vi "FitVItoLargestDecBounds.vi"(8 "error in (no error)":errorcluster, 11 "VI Ref (calling VI)":refnum<vi>) -> (0 "error out":errorcluster, 2 "content size":T1, 3 "dup VI Ref":refnum<vi>)   [LabVIEW 2021, in "TipStripOOPanelExample.lvlib" / "TipPanelExample.lvclass"]
uses:
  TipPanelExample.lvclass
  <vilib>/Utility/miscctls.llb/LVBoundsTypeDef.ctl
  TipPanelExample.lvclass/TipPanelExample.ctl
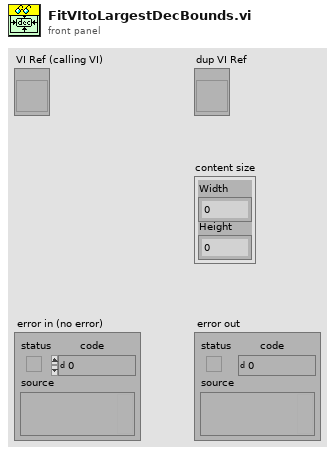
[diagram p1: front panel]
types:
  T1 = typedef "LVBoundsTypeDef.ctl" = cluster{"Width":u32, "Height":u32}
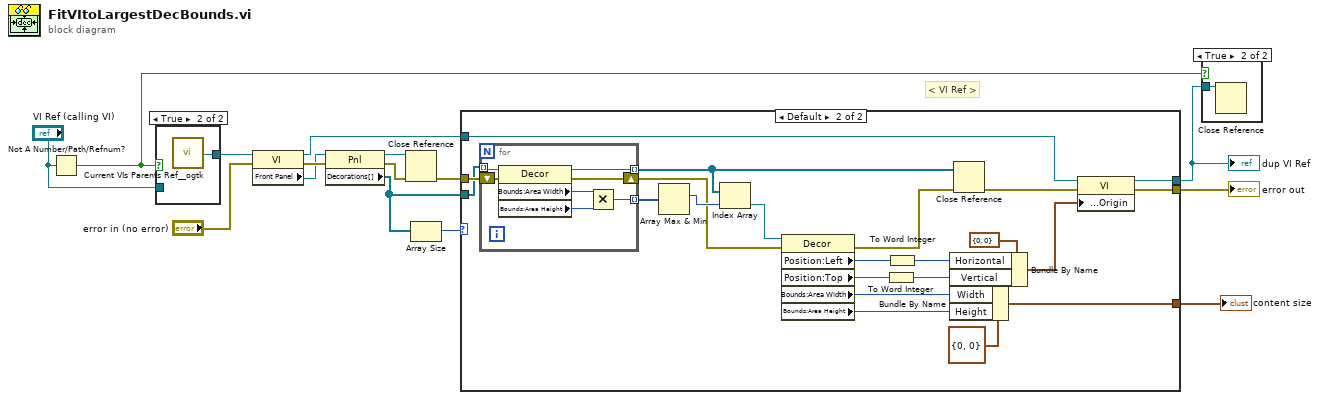
[diagram p0: block diagram]
diagram:
  # "< VI Ref >"
  n1 = Not A Number/Path/Refnum?(number/path/refnum="VI Ref (calling VI)") -> (NaN/Path/Refnum?=w3:bool)
  n2 = case shown="True" w3 {
    tunnel: [w16 w17] -> w4
    tunnel: "VI Ref (calling VI)" -> [w16 _]
    frame False {
    }
    frame True {
      n3 = call <userlib>:"Current VIs Parents Ref__ogtk.vi"() -> ("Calling VI's Reference"=w17:refnum<vi>)  [unwired: 2 in]
    }
  }
  n4 = property on="Property Node" class="VI"(reference=w4, error in="error in (no error)") -> (reference out=w15:refnum<vi>, error out=w13:errorcluster, "Front Panel"=w10:refnum<vi>)
  n5 = property on="Property Node" class="Pnl"(reference=w10, error in=w13) -> (reference out=w14:refnum<vi>, error out=w12:errorcluster, "Decorations[]"=w7:refnum<vi>[])
  n6 = Close Reference(reference=w14, error in (no error)=w12) -> (error out=w9:errorcluster)
  n7 = Array Size(array=w7) -> (size(s)=w6:i32)
  n8 = case shown="Default" w6 {
    tunnel: w15 -> [w19 w41]
    tunnel: w9 -> [w18 w36]
    tunnel: [w18 w24] -> w8
    tunnel: [w19 w25] -> w2
    tunnel: w7 -> [_ w28]
    tunnel: [_ w20] -> w1
    frame 0 {
    }
    frame Default {
      n9 = for {
        tunnel: w28 -> [w48] mode=indexing
        tunnel: [w45] -> w35 mode=indexing
        shift-right: [w43] -> w31
        shift-left: w36 -> [w44]
        tunnel: [w42] -> w33 mode=indexing
        n10 = property class="Decor"(reference=w48, error in=w44) -> (reference out=w42:refnum<vi>, error out=w43:errorcluster, "Bounds:Area Width"=w47:u32, "Bounds:Area Height"=w46:u32)
        n11 = Multiply(x=w47, y=w46) -> (x*y=w45:u32)
      }
      n12 = Array Max & Min(array=w35) -> (max index (indices)=w34:i32)  [unwired: 3 out]
      n13 = Index Array(array=w33, index=w34) -> (element=w32:refnum<vi>)
      n14 = property class="Decor"(reference=w32, error in=w31) -> (error out=w30:errorcluster, "Position:Left"=w39:i32, "Position:Top"=w40:i32, "Bounds:Area Width"=w22:u32, "Bounds:Area Height"=w21:u32)  [unwired: 1 out]
      n15 = To Word Integer(number=w40) -> (16bit integer=w27:i16)
      n16 = To Word Integer(number=w39) -> (16bit integer=w26:i16)
      n17 = Bundle By Name(cluster=cluster{"Horizontal":i16, "Vertical":i16} {"Horizontal"=0, "Vertical"=0} ("Front Panel Window:Origin"), "Horizontal"=w26, "Vertical"=w27) -> (w37:cluster{"Horizontal":i16, "Vertical":i16})
      n18 = Bundle By Name(cluster=T1 {"Width"=0, "Height"=0} ("content size"), "Width"=w22, "Height"=w21) -> (w20:T1)
      n19 = Close Reference(reference=w33, error in (no error)=w30) -> (error out=w29:errorcluster)
      n20 = property on="Property Node" class="VI"(reference=w41, error in=w29, "Front Panel Window:Origin"=w37) -> (reference out=w25:refnum<vi>, error out=w24:errorcluster)
    }
  }
  "error out" <- w8
  "dup VI Ref" <- w2
  "content size" <- w1
  n21 = case shown="True" w3 {
    tunnel: w2 -> [_ w49]
    frame False {
    }
    frame True {
      n22 = Close Reference(reference=w49) -> ()  [unwired: 1 in, 1 out]
    }
  }
